vi "RunBD.vi"(0 "VI refnum in":refnum<vi>, 5 "Wait until VI done?":bool caption="Wait until VI done? (F)", 7 "Auto dispose VI refnum?":bool=TRUE caption="Auto dispose VI refnum? (T)", 9 "Input data timeout":i32=-1 caption="Input data timeout (-1) [ms]" min=-1, 11 "Error in":errorcluster caption="Error in (no error)", 12 "Input data names":string[](array[string]) caption="Input data names (none)", 13 "Input data values":variant[](array[variant]) caption="Input data values (none)") -> (4 "VI refnum out":refnum<vi>, 6 "VI running?":bool, 8 "Last execution state":T1(ring), 10 "Input data timed out?":bool, 14 "Input data delivered?":bool, 15 "Error out":errorcluster)   [LabVIEW 2017, in "VILauncher.lvlib"]
doc: "Runs the dynamic VI specified by <B>VI refnum in</B>.\n\nThis function will wait until the dynamic VI is done if <B>Wait until VI done?</B> is True (default is False), and it will auto dispose the dynamic VI reference (hand it over to the running dynamic VI) if <B>Auto dispose VI refnum?</B> is True. Note that if this function fails to run the VI, <B>VI refnum in</B> will not be auto-disposed, in which case you retain the responsibility of closing that reference yourself.\n\nThe <B>VI running?</B> output will only be True if the dynamic VI's <B>Last execution state</B> is \"Run top level\". <B>VI running?</B> can be False even if the dynamic VI ran successfully - it might just have finished before this VI finished.\n\nOptionally you can send input data to the dynamic VI when running it using one of two modes; Right click this VI and use the Select Type menu to choose input data transfer mode:\n\nInput data via front panel\n-------------------------------\nSet data on the front panel of the dynamic VI before running it by wiring <B>Control names</B> and <B>Control values</B>. <B>Control values set?</B> will be True only if all <B>Control names</B> were valid.\n\nInput data via block diagram\n----------------------------------\nTransmit data to the dynamic VI after it has started by wiring <B>Input data names</B> and <B>Input data values</B>. If you use this mode the dynamic VI must use the WaitForInputData function to read the input data on the block diagram. The read in the dynamic VI must be finished before <B>Input data timeout</B> runs out. Set this timeout value to -1 (default) to wait indefinitely. If timeout does occur, <B>Input data timed out?</B> will be True. <B>Input data delivered?</B> will be True only if input data was in fact transmitted to the dynamic VI without any errors.\n\n<B>NOTE 1:</B> When using the 'Input data via block diagram' mode the dynamic VI must use the WaitForInputData function even if you send zero input data. To avoid this requirement for the dynamic VI when not passing any input data, please use the 'Input data via front panel' mode in this case.\n\n<B>NOTE 2:</B> The dynamic VI must have its front panel available at runtime for this function to work. The simplest way to ensure this, which also works in a built application without additional steps to be taken, is by enabling \"Show front panel when called\" in the \"Window Appearance\" section of the dynamic VI Properties.\n\nThis VI is reentrant, and it will run only if there is no error on <B>Error in</B>.\n\nSteen Schmidt\nGPower\n16/12 2013"
uses:
  VILauncher.lvlib
  Error/GPError.lvlib
  Timing/GPTiming.lvlib
  Timing/Library/Wait/Wait_ms.vi
  Timing/Library/Remaining/Remaining_ms.vi
panel:
  # "Copyright © 2013\nGPower\nSee enclosed license file for terms and conditions"
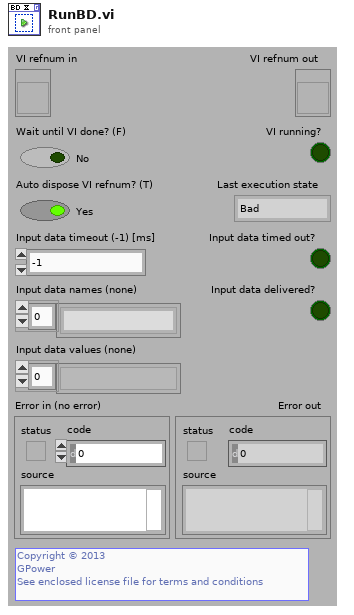
[diagram p1: front panel]
types:
  T1 = enum32{"Bad", "Idle", "Run top level", "Running"}
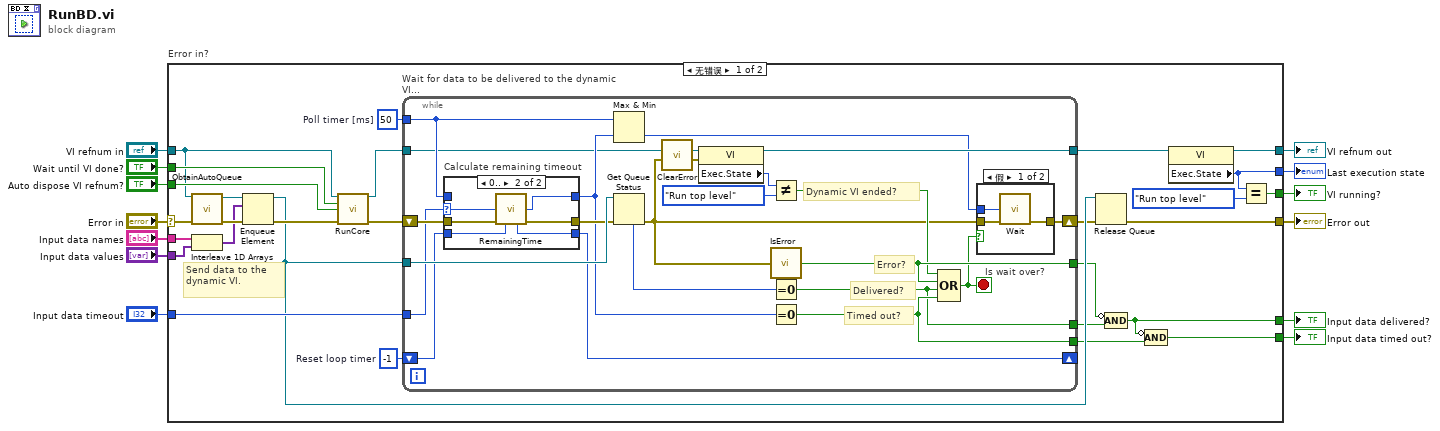
[diagram p0: block diagram]
diagram:
  n1 = case "Error in?" shown="无错误" "Error in" {
    selector: "Error in" -> [w21 w78]
    tunnel: [w41 _] -> w13
    tunnel: [w40 w77] -> w12
    tunnel: [w39 _] -> w11
    tunnel: [w37 _] -> w10
    tunnel: [w36 _] -> w9
    tunnel: "Input data names" -> [w35 _]
    tunnel: "Input data values" -> [w34 _]
    tunnel: "Wait until VI done?" -> [w32 _]
    tunnel: "VI refnum in" -> [w20 w77]
    tunnel: "Auto dispose VI refnum?" -> [w31 _]
    tunnel: "Input data timeout" -> [w29 _]
    tunnel: [w22 w78] -> w2
    frame No Error {
      w14 = i64 -1  # Reset loop timer
      w15 = 50  # Poll timer [ms]
      # "Send data to the\ndynamic VI."
      n2 = call "ObtainAutoQueue.vi"("VI reference in"=w20, "Error in"=w21) -> ("Queue"=w18:refnum<queue>, "Error out"=w19:errorcluster)  [unwired: 12 in]
      n3 = Interleave 1D Arrays(w35, w34) -> (w17:variant[])
      n4 = Enqueue Element(queue=w18, element=w17, error in (no error)=w19) -> (queue out=w28:refnum<queue>, error out=w33:errorcluster)  [unwired: 1 in, 1 out]
      n5 = call "RunCore.vi"("VI refnum in"=w20, "Wait until VI done?"=w32, "Auto dispose VI refnum?"=w31, "Error in"=w33) -> ("VI refnum out"=w24:refnum<vi>, "Error out"=w30:errorcluster)  [unwired: 8 in, 2 out]
      n6 = while "Wait for data to be delivered to the dynamic VI..." {
        shift-right: [w47] -> w16
        shift-left: w30 -> [w61]
        tunnel: w28 -> [w63]
        tunnel: w29 -> [w59]
        tunnel: [w58] -> w25
        tunnel: [w57] -> w26
        tunnel: [w49] -> w27
        tunnel: w15 -> [w55]
        tunnel: w24 -> [w52]
        tunnel: [w51] -> w23
        shift-right: [w44] -> _
        shift-left: w14 -> [w43]
        stop <- w45 stop-if-true
        # "Dynamic VI ended?"
        # "Error?"
        # "Delivered?"
        # "Timed out?"
        n7 = case "Calculate remaining timeout" shown="0.." w59 {
          selector: w59 -> [_ w73]
          tunnel: [w70 w76] -> w60
          tunnel: [w69 w72] -> w56
          tunnel: w43 -> [w68 w74]
          tunnel: w61 -> [w70 w75]
          tunnel: w55 -> [w69 _]
          tunnel: [w68 w71] -> w44
          frame ..-1 {
          }
          frame 0.. {
            n8 = call-poly "RemainingTime.vi"("Time period target"=w73, "Error in"=w75, "Start time in"=w74) -> ("Remaining time"=w72:i32, "Start time out"=w71:i64, "Error out"=w76:errorcluster)  [unwired: 8 in, 2 out]
          }
        }
        n9 = Max & Min(x=w55, y=w56) -> (min(x,y)=w46:i32)  [unwired: 1 out]
        n10 = Get Queue Status(queue=w63, error in (no error)=w60) -> (error out=w42:errorcluster, # elements in queue=w62:i32)  [unwired: 1 in, 6 out]
        n11 = call "ClearError.vi"("Error in"=w42) -> ("Error out"=w50:errorcluster)  [unwired: 10 in]
        n12 = property class="VI"(reference=w52, error in=w50) -> (reference out=w51:refnum<vi>, "Exec.State"=w54:T1)  [unwired: 1 out]
        n13 = Not Equal?(x=w54, y=T1."Run top level") -> (x != y?=w48:bool)
        n14 = call "IsError.vi"("Error in"=w42) -> ("Error?"=w49:bool)  [unwired: 4 in]
        n15 = Equal To 0?(x=w62) -> (x = 0?=w57:bool)
        n16 = Equal To 0?(x=w56) -> (x = 0?=w58:bool)
        n17 = Compound Arithmetic op=OR(w48, w49, w57, w58) -> (w45:bool)
        n18 = case "Is wait over?" shown="假" w45 {
          tunnel: [w66 w67] -> w47
          tunnel: w42 -> [w65 w67]
          tunnel: w46 -> [w64 _]
          frame False {
            n19 = call-poly "Wait.vi"("Time to wait"=w64, "Error in"=w65) -> ("Error out"=w66:errorcluster)  [unwired: 13 in]
          }
          frame True {
          }
        }
      }
      n20 = Release Queue(queue=w28, error in (no error)=w16) -> (error out=w22:errorcluster)  [unwired: 1 in, 2 out]
      n21 = Compound Arithmetic op=AND(invert w27, w26) -> (w36:bool)
      n22 = Compound Arithmetic op=AND(invert w36, w25) -> (w37:bool)
      n23 = property class="VI"(reference=w23) -> (reference out=w40:refnum<vi>, "Exec.State"=w39:T1)  [unwired: 1 in, 1 out]
      n24 = Equal?(x=w39, y=T1."Run top level") -> (x = y?=w41:bool)
    }
    frame Error {
    }
  }
  "Error out" <- w2
  "VI refnum out" <- w12
  "VI running?" <- w13
  "Last execution state" <- w11
  "Input data timed out?" <- w10
  "Input data delivered?" <- w9
